vi "FluorimeterReadoutUpdatedLaptop.vi"() -> ()   [LabVIEW 2018]
uses:
  <vilib>/Utility/file.llb/Write Delimited Spreadsheet (DBL).vi
panel:
  out "Readout":dbl
  out "?":dbl(graph)
  in  "?":bool
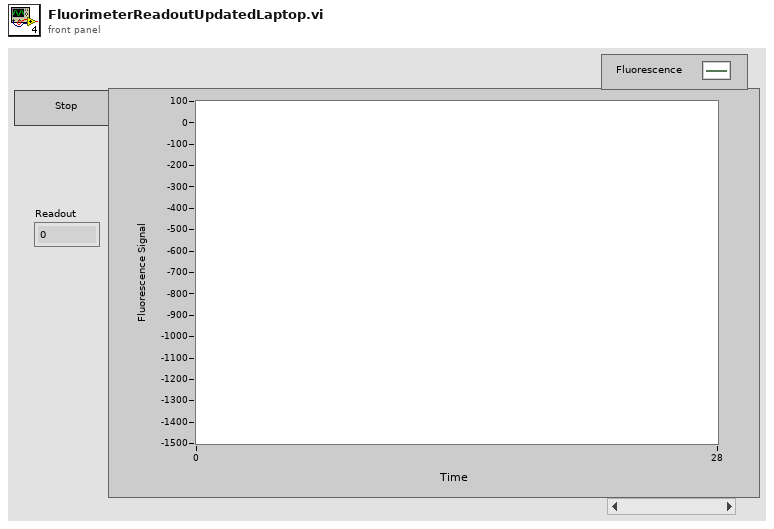
[diagram p1: front panel]
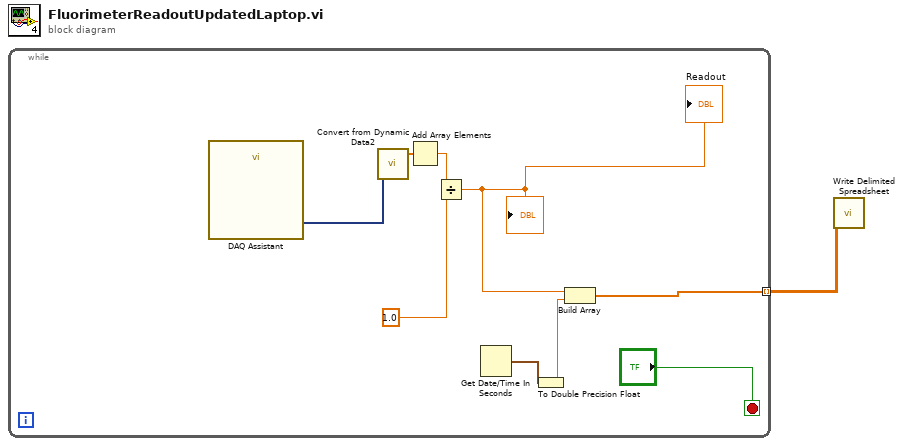
[diagram p0: block diagram]
diagram:
  n1 = while {
    tunnel: [w3] -> w1 mode=indexing
    stop <- "?" stop-if-true
    n2 = call "DAQ Assistant"() -> ("data"=w2:dynamicdata)  [unwired: 16 in, 3 out]
    n3 = call "Convert from Dynamic Data2"("Dynamic Data Type"=w2) -> ("Array"=w9:dbl[])  [unwired: 3 in]
    n4 = Add Array Elements(numeric array=w9) -> (sum=w7:dbl)
    n5 = Divide(x=w7, y=1.0) -> (x/y=w6:dbl)
    "?" <- w6
    "Readout" <- w6
    n6 = Get Date/Time In Seconds() -> (seconds since 1Jan1904=w5:timestamp)
    n7 = To Double Precision Float(number=w5) -> (double precision float=w4:dbl)
    n8 = Build Array(w6, w4) -> (w3:dbl[])
  }
  n9 = call-poly <vilib>:"Write Delimited Spreadsheet.vi"("2D data"=w1) -> ()  [unwired: 13 in, 2 out]
